vi "Train Approach.vi"(3 "Cycle State In":T1) -> (0 "Cycle State Out":T1)   [LabVIEW 2020]
uses:
  Reset.ctl
  Cycle Status.ctl
  Cycle Enum.ctl
  Grade Gate.ctl
  Global Indicators.vi
panel:
  out "Cycle Status":T2
  in  "Reset":T3
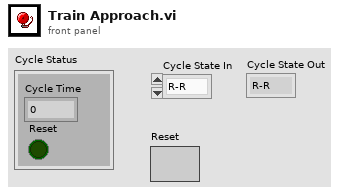
[diagram p1: front panel]
types:
  T1 = typedef "Cycle Enum.ctl" = enum16{"R-R", "NS Left G", "NS Left Y", "NS Straight G", "NS Straight Y", "r-r", "WE Left G", "WE Left Y", "WE Straight G", "WE Straight Y", "N All G", "S All G", "W All G", "E All G", "Gate Up", "Gate Mid", "Blink 1", "End Train", "Blink 2"}
  T2 = typedef "Cycle Status.ctl" = cluster{"Cycle Time":dbl, "Reset":bool}
  T3 = typedef "Reset.ctl" = bool
  T4 = typedef "Grade Gate.ctl" = cluster{"UP 2":bool, "Pivot":bool, "UP 3":bool, "UP 4":bool, "UP 5":bool, "UP 6":bool, "DOWN 2":bool, "DOWN 3":bool, "DOWN 4":bool, "DOWN 5":bool, "DOWN 6":bool, "DOWN 7":bool, "DOWN 8":bool, "SIDE 2":bool, "SIDE 3":bool, "SIDE 4":bool, "SIDE 5":bool, "Blinky 2":bool, "Blinky 1":bool}
  T5 = typedef "Traffic Signal.ctl" = cluster{"Red Light":bool, "Yellow Light":bool, "Green Light":bool, "Yellow Turn":bool, "Green Turn":bool}
  T6 = typedef "PedX Signal.ctl" = cluster{"PedX Walk":bool, "PedX Stop":bool}
  T7 = enum16{"R-R", "NS Left G", "NS Left Y", "NS Straight G", "NS Straight Y", "r-r", "WE Left G", "WE Left Y", "WE Straight G", "WE Straight Y"}
  T8 = enum16{"R-R", "NS Left G", "NS Left Y", "NS Straight G", "NS Straight Y"}
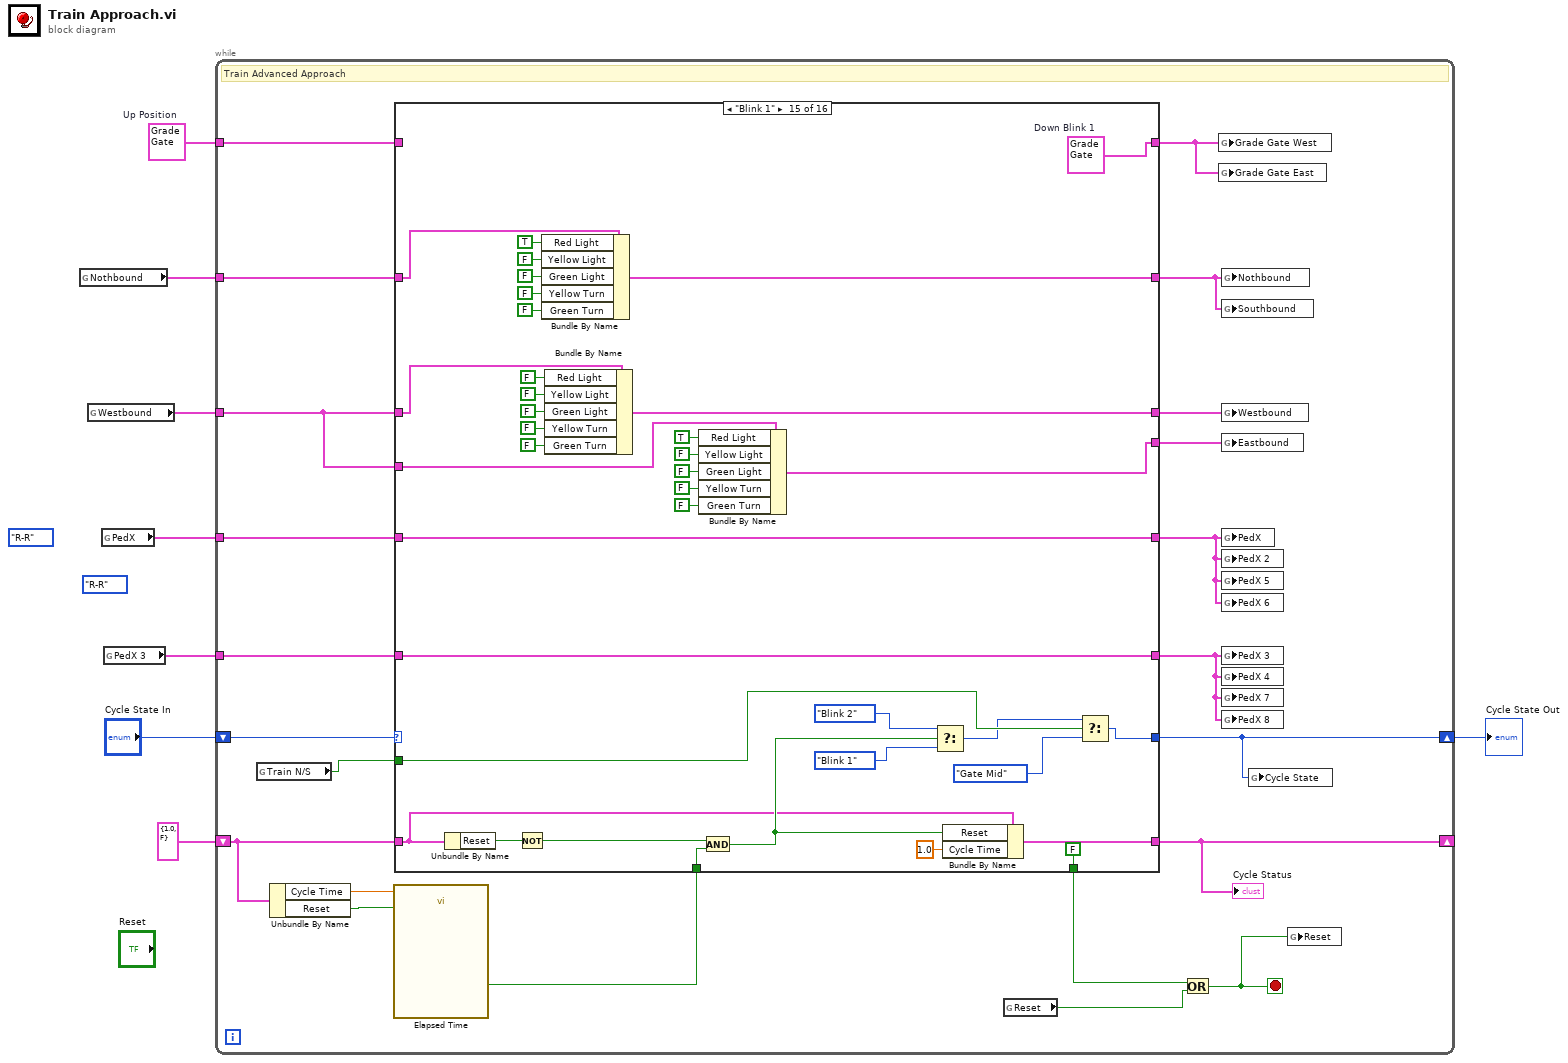
[diagram p0: block diagram]
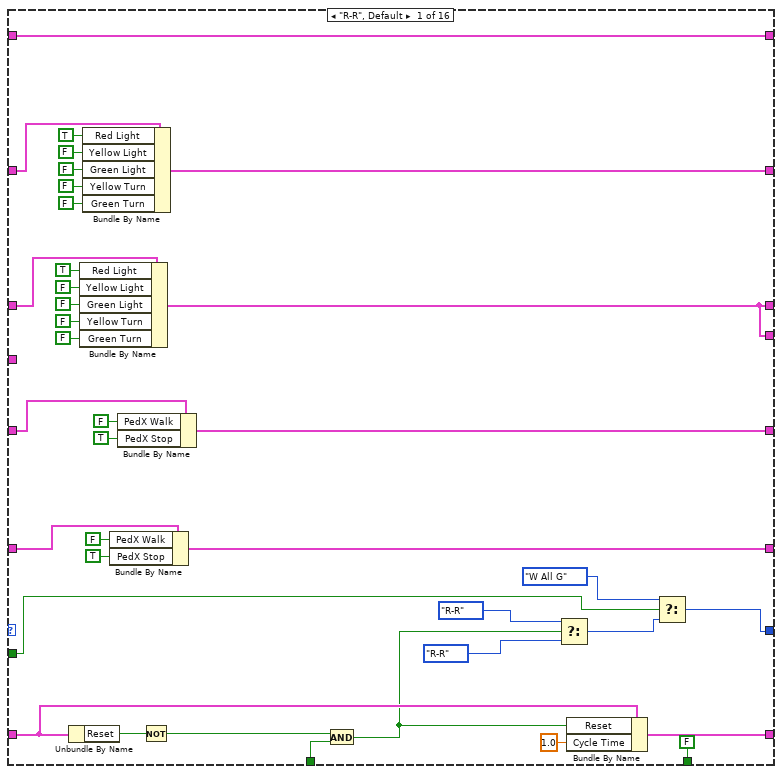
[diagram p2: hidden frame]
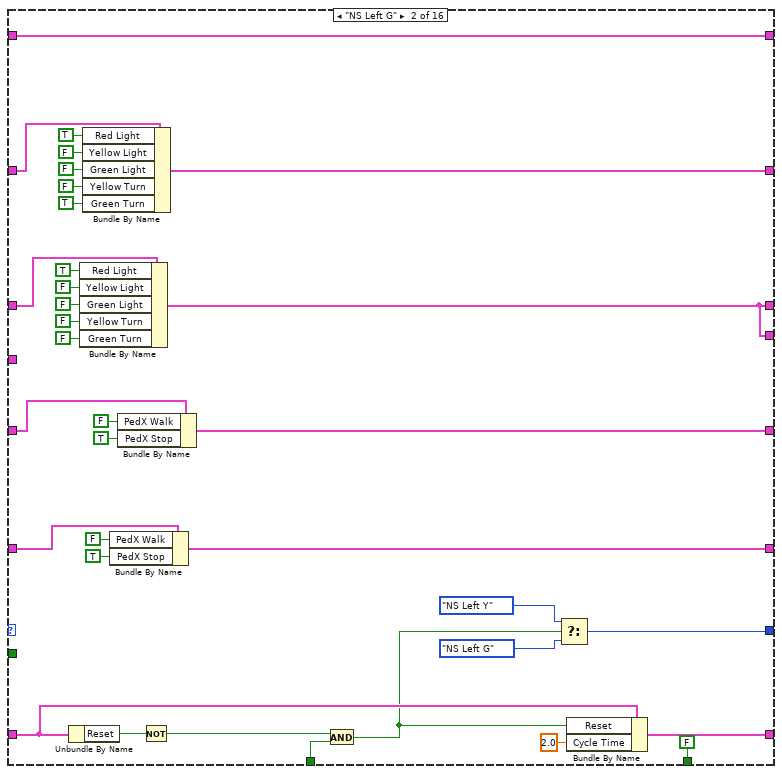
[diagram p3: hidden frame]
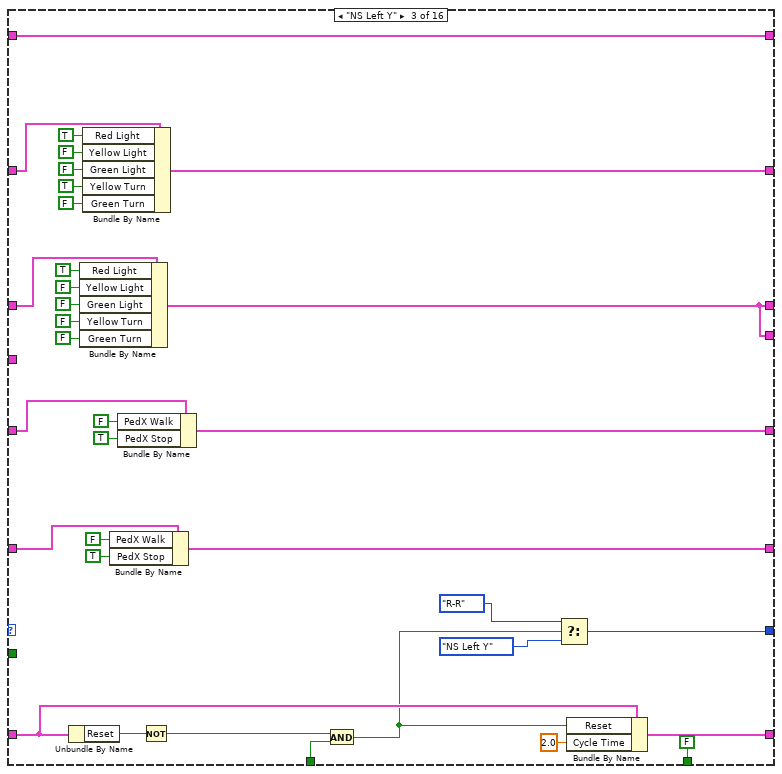
[diagram p4: hidden frame]
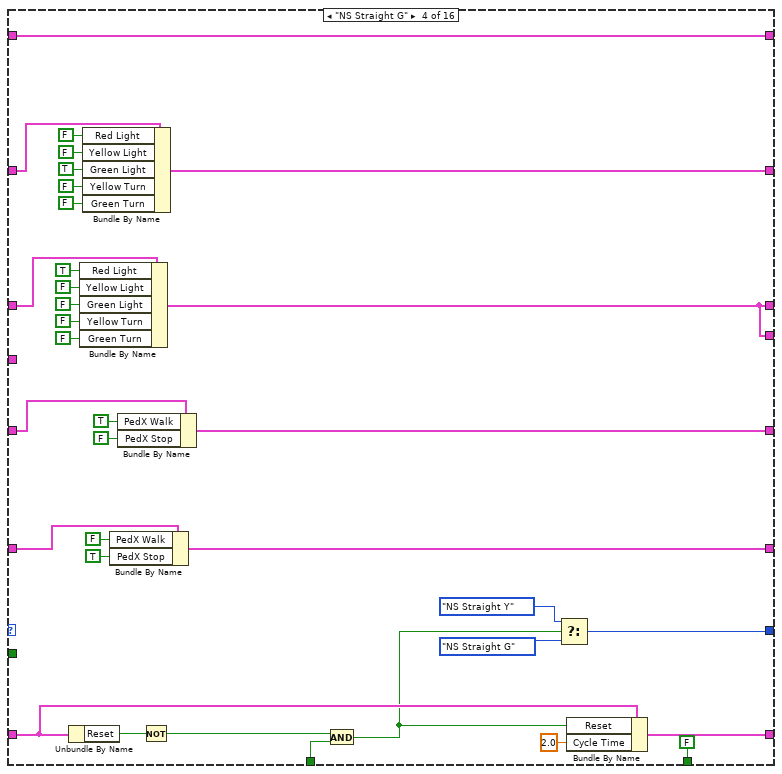
[diagram p5: hidden frame]
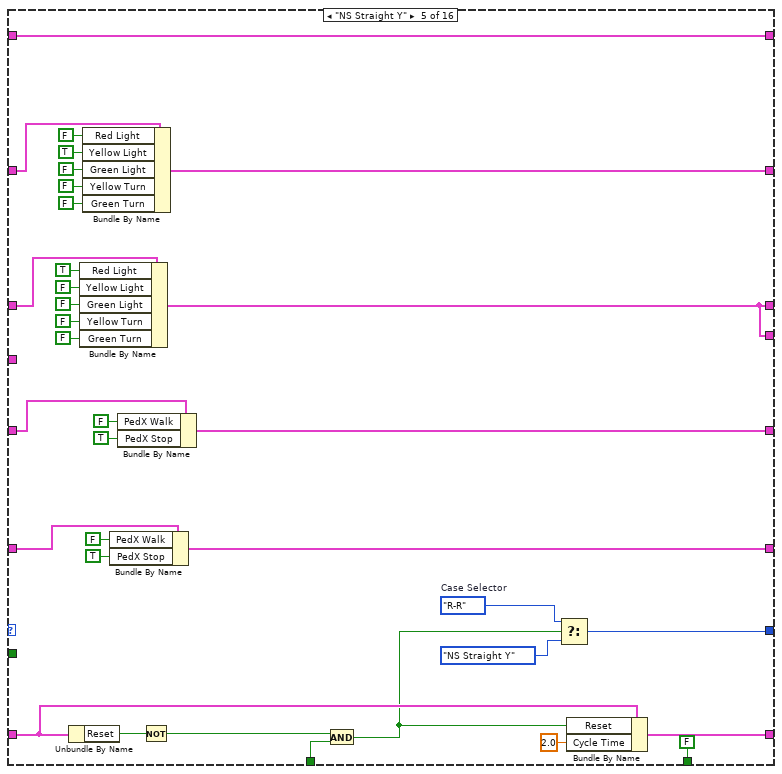
[diagram p6: hidden frame]
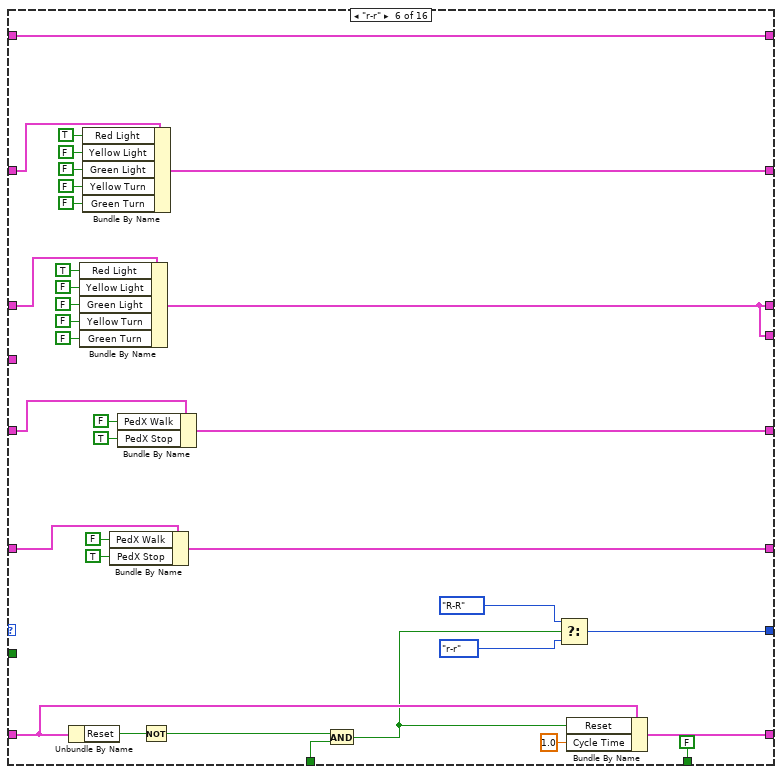
[diagram p7: hidden frame]
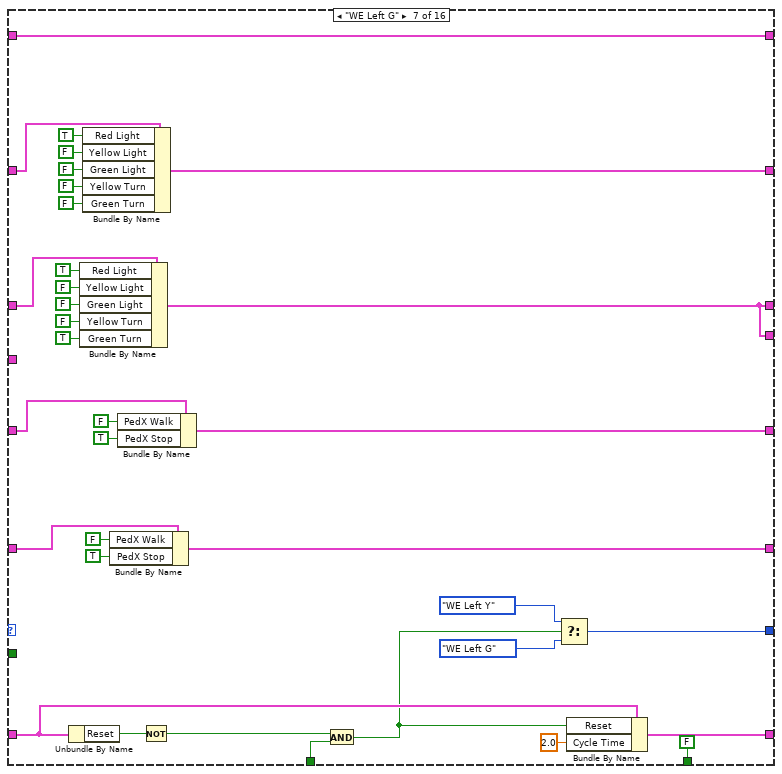
[diagram p8: hidden frame]
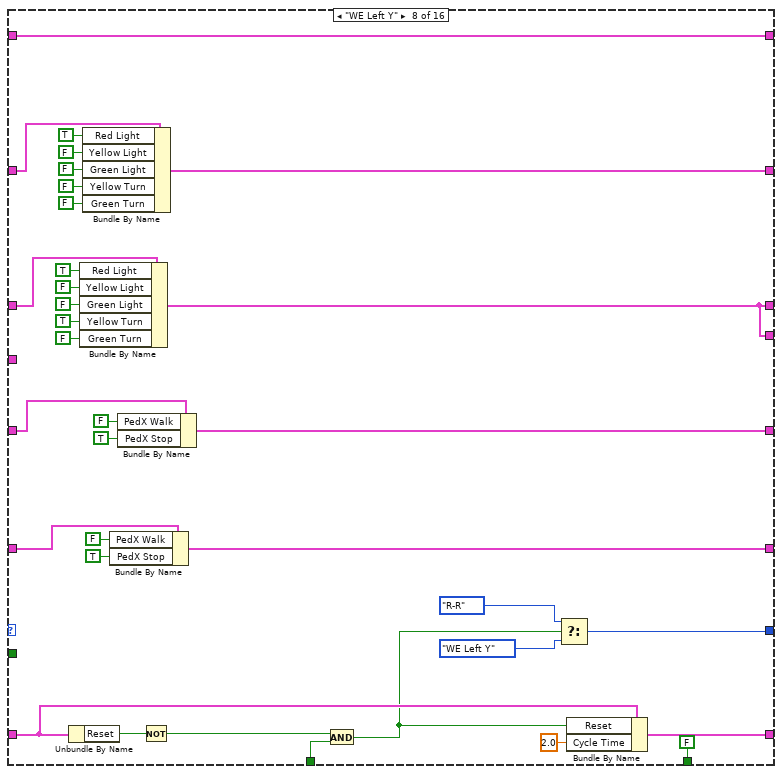
[diagram p9: hidden frame]
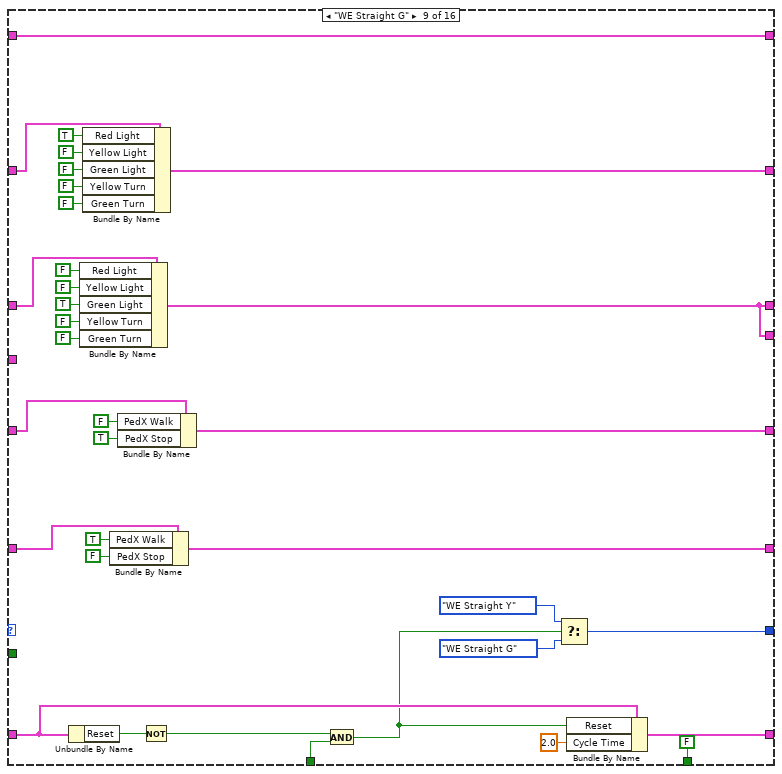
[diagram p10: hidden frame]
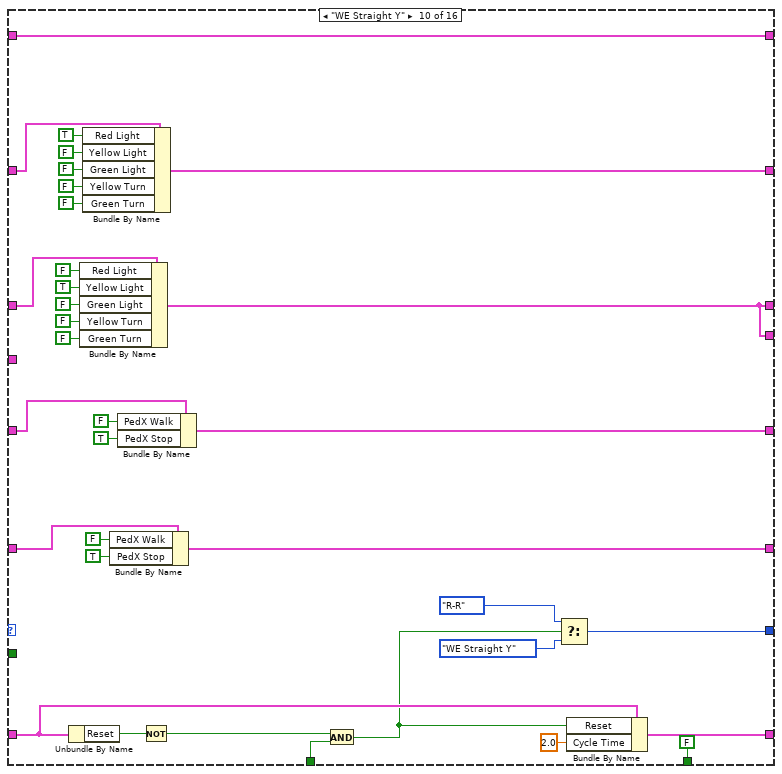
[diagram p11: hidden frame]
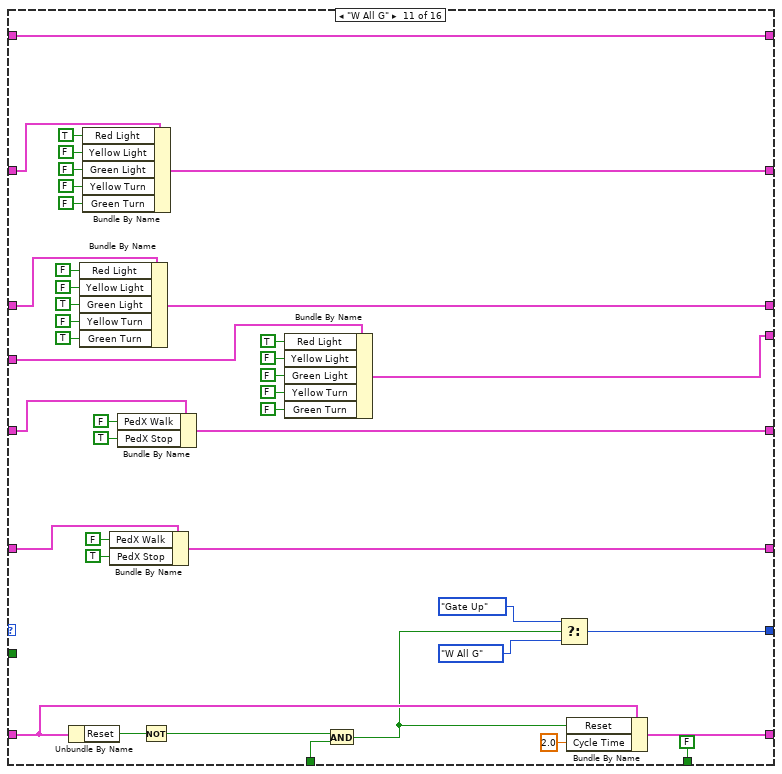
[diagram p12: hidden frame]
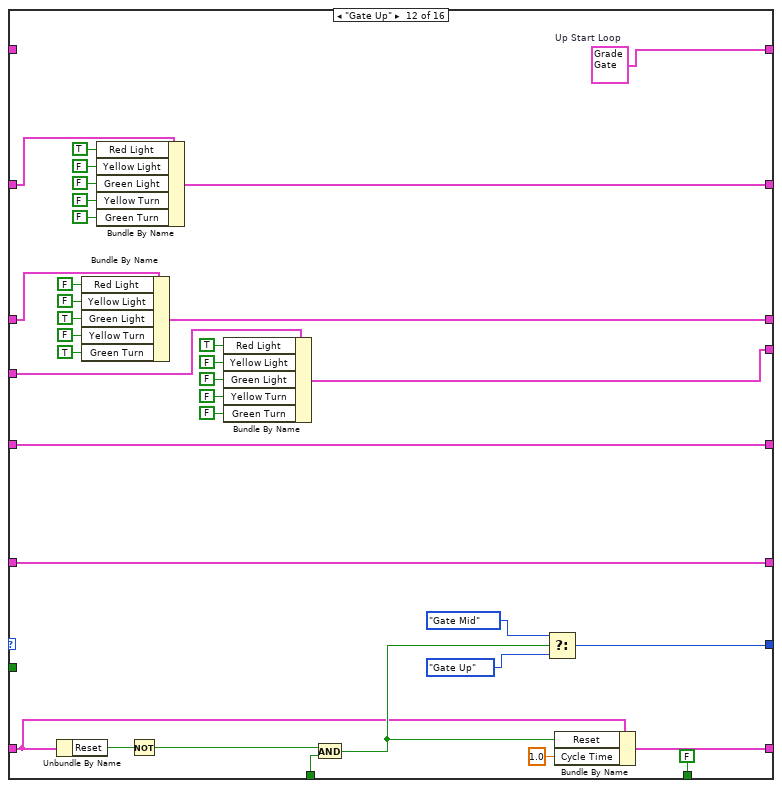
[diagram p13: hidden frame]
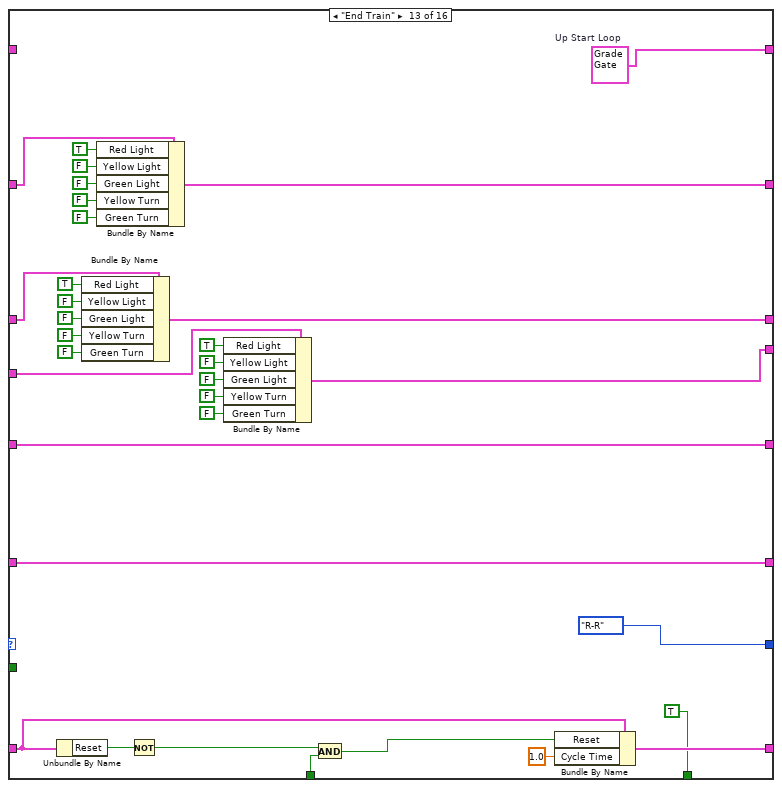
[diagram p14: hidden frame]
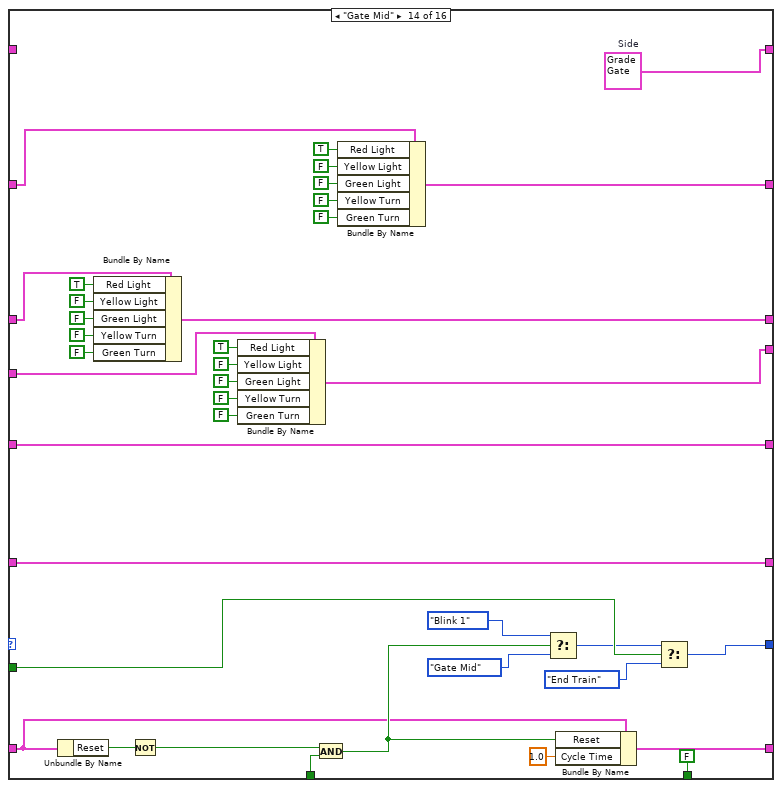
[diagram p15: hidden frame]
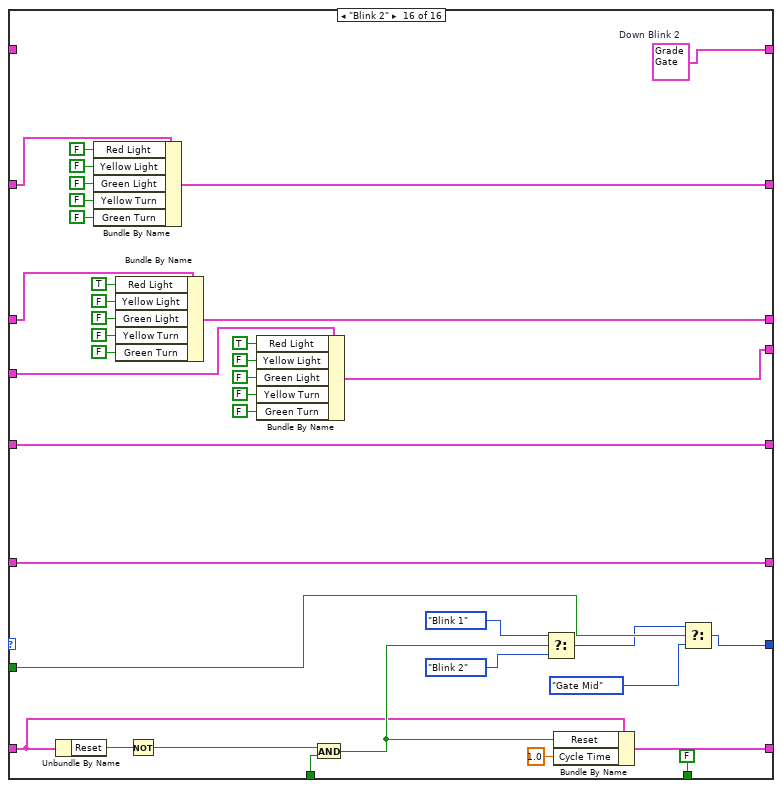
[diagram p16: hidden frame]
diagram:
  (unwired) Cycle_Enum."R-R" ("Cycle State In")
  (unwired) Cycle_Enum."R-R" ("Cycle State In")
  w8 = T4 {"UP 2"=FALSE, "Pivot"=FALSE, "UP 3"=TRUE, "UP 4"=FALSE, "UP 5"=FALSE, "UP 6"=FALSE, "DOWN 2"=FALSE, "DOWN 3"=FALSE, "DOWN 4"=FALSE, "DOWN 5"=FALSE, "DOWN 6"=FALSE, "DOWN 7"=FALSE, "DOWN 8"=FALSE, "SIDE 2"=FALSE, "SIDE 3"=FALSE, "SIDE 4"=FALSE, "SIDE 5"=FALSE, "Blinky 2"=FALSE, "Blinky 1"=FALSE}  # Up Position
  n1 = global read "Global Indicators.vi" "Nothbound"() -> (w6:T5)
  n2 = global read "Global Indicators.vi" "Westbound"() -> (w5:T5)
  n3 = global read "Global Indicators.vi" "PedX"() -> (w4:T6)
  n4 = global read "Global Indicators.vi" "PedX 3"() -> (w3:T6)
  n5 = while {
    shift-right: [w15] -> w1
    shift-left: "Cycle State In" -> [w17]
    tunnel: w8 -> [w26]
    tunnel: w5 -> [w14]
    tunnel: w6 -> [w25]
    tunnel: w4 -> [w24]
    tunnel: w3 -> [w23]
    shift-right: [w16] -> _
    shift-left: T2 {"Cycle Time"=1.0, "Reset"=FALSE} ("Cycle Status") -> [w22]
    stop <- w9 stop-if-true
    # "Train Advanced Approach"
    n6 = global read "Global Indicators.vi" "Train N/S"() -> (w10:bool)
    n7 = Unbundle By Name(w22) -> ("Cycle Time"=w30:dbl, "Reset"=w29:bool)
    n8 = call "Elapsed Time"("Time Target (s)"=w30, "Reset"=w29) -> ("Time has Elapsed"=w28:bool)  [unwired: 10 in, 7 out]
    n9 = case shown="\"Blink 1\"" w17 {
      tunnel: [w67 w101 w135 w169 w203 w237 w271 w305 w339 w373 w414 w449 w482 w520 w558 w596] -> w27
      tunnel: w26 -> [w67 w101 w135 w169 w203 w237 w271 w305 w339 w373 w414 _ _ _ _ _]
      tunnel: [w60 w94 w128 w162 w196 w230 w264 w298 w332 w366 w407 w445 w478 w518 w556 w592] -> w21
      tunnel: w25 -> [w66 w100 w134 w168 w202 w236 w270 w304 w338 w372 w413 w446 w479 w519 w557 w593]
      tunnel: [w37 w69 w103 w137 w171 w205 w239 w273 w307 w341 w393 w438 w471 w511 w549 w585] -> w20
      tunnel: w14 -> [w48 w81 w114 w147 w183 w217 w251 w285 w319 w353 w394 w439 w472 w512 w550 w586]
      tunnel: [w56 w90 w124 w158 w192 w226 w260 w294 w328 w362 w403 w448 w481 w505 w543 w595] -> w19
      tunnel: w24 -> [w59 w93 w127 w161 w195 w229 w263 w297 w331 w365 w406 w448 w481 w505 w543 w595]
      tunnel: w23 -> [w39 w72 w105 w138 w174 w208 w242 w276 w310 w344 w384 w447 w480 w504 w542 w594]
      tunnel: [w40 w73 w106 w139 w175 w209 w243 w277 w311 w345 w385 w447 w480 w504 w542 w594] -> w18
      tunnel: [w52 w85 w118 w151 w187 w221 w255 w289 w323 w357 w398 w418 w454 w490 w528 w566] -> w16
      tunnel: w22 -> [w51 w84 w117 w150 w186 w220 w254 w288 w322 w356 w397 w417 w453 w489 w527 w565]
      tunnel: [w33 w86 w120 w154 w188 w222 w256 w290 w324 w358 w399 w419 Cycle_Enum."R-R" ("Cycle State In") w487 w525 w562] -> w15
      tunnel: w28 -> [w53 w87 w121 w155 w189 w223 w257 w291 w325 w359 w400 w416 w452 w488 w526 w564]
      tunnel: w14 -> [_ _ _ _ _ _ _ _ _ _ w383 w432 w465 w503 w541 w579]
      tunnel: [w37 w69 w103 w137 w171 w205 w239 w273 w307 w341 w377 w431 w464 w502 w540 w578] -> w13
      tunnel: w10 -> [w32 _ _ _ _ _ _ _ _ _ _ _ _ w486 w524 w563]
      tunnel: [FALSE FALSE FALSE FALSE FALSE FALSE FALSE FALSE FALSE FALSE FALSE FALSE TRUE FALSE FALSE FALSE] -> w11
      frame "R-R", Default {
        n10 = Unbundle By Name(w51) -> ("Reset"=w55:bool)
        n11 = Bundle By Name(cluster=w48, "Red Light"=TRUE, "Yellow Light"=FALSE, "Green Light"=FALSE, "Yellow Turn"=FALSE, "Green Turn"=FALSE) -> (w37:T5)
        n12 = Bundle By Name(cluster=w66, "Red Light"=TRUE, "Yellow Light"=FALSE, "Green Light"=FALSE, "Yellow Turn"=FALSE, "Green Turn"=FALSE) -> (w60:T5)
        n13 = Bundle By Name(cluster=w39, "PedX Walk"=FALSE, "PedX Stop"=TRUE) -> (w40:T6)
        n14 = Bundle By Name(cluster=w59, "PedX Walk"=FALSE, "PedX Stop"=TRUE) -> (w56:T6)
        n15 = Not(x=w55) -> (.not. x?=w54:bool)
        n16 = And(x=w54, y=w53) -> (x .and. y?=w50:bool)
        n17 = Select(t=Cycle_Enum."R-R" ("Cycle State In"), s=w50, f=Cycle_Enum."R-R" ("Cycle State In")) -> (s? t:f=w34:T1)
        n18 = Bundle By Name(cluster=w51, "Reset"=w50, "Cycle Time"=1.0) -> (w52:T2)
        n19 = Select(t=Cycle_Enum."W All G" ("Cycle State In"), s=w32, f=w34) -> (s? t:f=w33:T1)
      }
      frame "NS Left G" {
        n20 = Unbundle By Name(w84) -> ("Reset"=w89:bool)
        n21 = Bundle By Name(cluster=w81, "Red Light"=TRUE, "Yellow Light"=FALSE, "Green Light"=FALSE, "Yellow Turn"=FALSE, "Green Turn"=FALSE) -> (w69:T5)
        n22 = Bundle By Name(cluster=w100, "Red Light"=TRUE, "Yellow Light"=FALSE, "Green Light"=FALSE, "Yellow Turn"=FALSE, "Green Turn"=TRUE) -> (w94:T5)
        n23 = Bundle By Name(cluster=w72, "PedX Walk"=FALSE, "PedX Stop"=TRUE) -> (w73:T6)
        n24 = Bundle By Name(cluster=w93, "PedX Walk"=FALSE, "PedX Stop"=TRUE) -> (w90:T6)
        n25 = Not(x=w89) -> (.not. x?=w88:bool)
        n26 = And(x=w88, y=w87) -> (x .and. y?=w83:bool)
        n27 = Select(t=T7."NS Left Y" ("Case Selector"), s=w83, f=T7."NS Left G" ("Case Selector")) -> (s? t:f=w86:T7)
        n28 = Bundle By Name(cluster=w84, "Reset"=w83, "Cycle Time"=2.0) -> (w85:T2)
      }
      frame "NS Left Y" {
        n29 = Unbundle By Name(w117) -> ("Reset"=w123:bool)
        n30 = Bundle By Name(cluster=w114, "Red Light"=TRUE, "Yellow Light"=FALSE, "Green Light"=FALSE, "Yellow Turn"=FALSE, "Green Turn"=FALSE) -> (w103:T5)
        n31 = Bundle By Name(cluster=w134, "Red Light"=TRUE, "Yellow Light"=FALSE, "Green Light"=FALSE, "Yellow Turn"=TRUE, "Green Turn"=FALSE) -> (w128:T5)
        n32 = Bundle By Name(cluster=w105, "PedX Walk"=FALSE, "PedX Stop"=TRUE) -> (w106:T6)
        n33 = Bundle By Name(cluster=w127, "PedX Walk"=FALSE, "PedX Stop"=TRUE) -> (w124:T6)
        n34 = Not(x=w123) -> (.not. x?=w122:bool)
        n35 = And(x=w122, y=w121) -> (x .and. y?=w116:bool)
        n36 = Select(t=Cycle_Enum."R-R" ("Cycle State In"), s=w116, f=T8."NS Left Y" ("Case Selector")) -> (s? t:f=w120:T1)
        n37 = Bundle By Name(cluster=w117, "Reset"=w116, "Cycle Time"=2.0) -> (w118:T2)
      }
      frame "NS Straight G" {
        n38 = Unbundle By Name(w150) -> ("Reset"=w157:bool)
        n39 = Bundle By Name(cluster=w147, "Red Light"=TRUE, "Yellow Light"=FALSE, "Green Light"=FALSE, "Yellow Turn"=FALSE, "Green Turn"=FALSE) -> (w137:T5)
        n40 = Bundle By Name(cluster=w168, "Red Light"=FALSE, "Yellow Light"=FALSE, "Green Light"=TRUE, "Yellow Turn"=FALSE, "Green Turn"=FALSE) -> (w162:T5)
        n41 = Bundle By Name(cluster=w138, "PedX Walk"=FALSE, "PedX Stop"=TRUE) -> (w139:T6)
        n42 = Bundle By Name(cluster=w161, "PedX Walk"=TRUE, "PedX Stop"=FALSE) -> (w158:T6)
        n43 = Not(x=w157) -> (.not. x?=w156:bool)
        n44 = And(x=w156, y=w155) -> (x .and. y?=w149:bool)
        n45 = Select(t=T8."NS Straight Y" ("Case Selector"), s=w149, f=T8."NS Straight G" ("Case Selector")) -> (s? t:f=w154:T8)
        n46 = Bundle By Name(cluster=w150, "Reset"=w149, "Cycle Time"=2.0) -> (w151:T2)
      }
      frame "NS Straight Y" {
        w173 = T7."R-R"  # Case Selector
        n47 = Unbundle By Name(w186) -> ("Reset"=w191:bool)
        n48 = Bundle By Name(cluster=w183, "Red Light"=TRUE, "Yellow Light"=FALSE, "Green Light"=FALSE, "Yellow Turn"=FALSE, "Green Turn"=FALSE) -> (w171:T5)
        n49 = Bundle By Name(cluster=w202, "Red Light"=FALSE, "Yellow Light"=TRUE, "Green Light"=FALSE, "Yellow Turn"=FALSE, "Green Turn"=FALSE) -> (w196:T5)
        n50 = Bundle By Name(cluster=w174, "PedX Walk"=FALSE, "PedX Stop"=TRUE) -> (w175:T6)
        n51 = Bundle By Name(cluster=w195, "PedX Walk"=FALSE, "PedX Stop"=TRUE) -> (w192:T6)
        n52 = Not(x=w191) -> (.not. x?=w190:bool)
        n53 = And(x=w190, y=w189) -> (x .and. y?=w185:bool)
        n54 = Select(t=w173, s=w185, f=T7."NS Straight Y" ("Case Selector")) -> (s? t:f=w188:T7)
        n55 = Bundle By Name(cluster=w186, "Reset"=w185, "Cycle Time"=2.0) -> (w187:T2)
      }
      frame "r-r" {
        n56 = Unbundle By Name(w220) -> ("Reset"=w225:bool)
        n57 = Bundle By Name(cluster=w217, "Red Light"=TRUE, "Yellow Light"=FALSE, "Green Light"=FALSE, "Yellow Turn"=FALSE, "Green Turn"=FALSE) -> (w205:T5)
        n58 = Bundle By Name(cluster=w236, "Red Light"=TRUE, "Yellow Light"=FALSE, "Green Light"=FALSE, "Yellow Turn"=FALSE, "Green Turn"=FALSE) -> (w230:T5)
        n59 = Bundle By Name(cluster=w208, "PedX Walk"=FALSE, "PedX Stop"=TRUE) -> (w209:T6)
        n60 = Bundle By Name(cluster=w229, "PedX Walk"=FALSE, "PedX Stop"=TRUE) -> (w226:T6)
        n61 = Not(x=w225) -> (.not. x?=w224:bool)
        n62 = And(x=w224, y=w223) -> (x .and. y?=w219:bool)
        n63 = Select(t=T7."R-R" ("Case Selector"), s=w219, f=T7."r-r" ("Case Selector")) -> (s? t:f=w222:T7)
        n64 = Bundle By Name(cluster=w220, "Reset"=w219, "Cycle Time"=1.0) -> (w221:T2)
      }
      frame "WE Left G" {
        n65 = Unbundle By Name(w254) -> ("Reset"=w259:bool)
        n66 = Bundle By Name(cluster=w251, "Red Light"=TRUE, "Yellow Light"=FALSE, "Green Light"=FALSE, "Yellow Turn"=FALSE, "Green Turn"=TRUE) -> (w239:T5)
        n67 = Bundle By Name(cluster=w270, "Red Light"=TRUE, "Yellow Light"=FALSE, "Green Light"=FALSE, "Yellow Turn"=FALSE, "Green Turn"=FALSE) -> (w264:T5)
        n68 = Bundle By Name(cluster=w242, "PedX Walk"=FALSE, "PedX Stop"=TRUE) -> (w243:T6)
        n69 = Bundle By Name(cluster=w263, "PedX Walk"=FALSE, "PedX Stop"=TRUE) -> (w260:T6)
        n70 = Not(x=w259) -> (.not. x?=w258:bool)
        n71 = And(x=w258, y=w257) -> (x .and. y?=w253:bool)
        n72 = Select(t=T7."WE Left Y" ("Case Selector"), s=w253, f=T7."WE Left G" ("Case Selector")) -> (s? t:f=w256:T7)
        n73 = Bundle By Name(cluster=w254, "Reset"=w253, "Cycle Time"=2.0) -> (w255:T2)
      }
      frame "WE Left Y" {
        n74 = Unbundle By Name(w288) -> ("Reset"=w293:bool)
        n75 = Bundle By Name(cluster=w285, "Red Light"=TRUE, "Yellow Light"=FALSE, "Green Light"=FALSE, "Yellow Turn"=TRUE, "Green Turn"=FALSE) -> (w273:T5)
        n76 = Bundle By Name(cluster=w304, "Red Light"=TRUE, "Yellow Light"=FALSE, "Green Light"=FALSE, "Yellow Turn"=FALSE, "Green Turn"=FALSE) -> (w298:T5)
        n77 = Bundle By Name(cluster=w276, "PedX Walk"=FALSE, "PedX Stop"=TRUE) -> (w277:T6)
        n78 = Bundle By Name(cluster=w297, "PedX Walk"=FALSE, "PedX Stop"=TRUE) -> (w294:T6)
        n79 = Not(x=w293) -> (.not. x?=w292:bool)
        n80 = And(x=w292, y=w291) -> (x .and. y?=w287:bool)
        n81 = Select(t=T7."R-R" ("Case Selector"), s=w287, f=T7."WE Left Y" ("Case Selector")) -> (s? t:f=w290:T7)
        n82 = Bundle By Name(cluster=w288, "Reset"=w287, "Cycle Time"=2.0) -> (w289:T2)
      }
      frame "WE Straight G" {
        n83 = Unbundle By Name(w322) -> ("Reset"=w327:bool)
        n84 = Bundle By Name(cluster=w319, "Red Light"=FALSE, "Yellow Light"=FALSE, "Green Light"=TRUE, "Yellow Turn"=FALSE, "Green Turn"=FALSE) -> (w307:T5)
        n85 = Bundle By Name(cluster=w338, "Red Light"=TRUE, "Yellow Light"=FALSE, "Green Light"=FALSE, "Yellow Turn"=FALSE, "Green Turn"=FALSE) -> (w332:T5)
        n86 = Bundle By Name(cluster=w310, "PedX Walk"=TRUE, "PedX Stop"=FALSE) -> (w311:T6)
        n87 = Bundle By Name(cluster=w331, "PedX Walk"=FALSE, "PedX Stop"=TRUE) -> (w328:T6)
        n88 = Not(x=w327) -> (.not. x?=w326:bool)
        n89 = And(x=w326, y=w325) -> (x .and. y?=w321:bool)
        n90 = Select(t=T7."WE Straight Y" ("Case Selector"), s=w321, f=T7."WE Straight G" ("Case Selector")) -> (s? t:f=w324:T7)
        n91 = Bundle By Name(cluster=w322, "Reset"=w321, "Cycle Time"=2.0) -> (w323:T2)
      }
      frame "WE Straight Y" {
        n92 = Unbundle By Name(w356) -> ("Reset"=w361:bool)
        n93 = Bundle By Name(cluster=w353, "Red Light"=FALSE, "Yellow Light"=TRUE, "Green Light"=FALSE, "Yellow Turn"=FALSE, "Green Turn"=FALSE) -> (w341:T5)
        n94 = Bundle By Name(cluster=w372, "Red Light"=TRUE, "Yellow Light"=FALSE, "Green Light"=FALSE, "Yellow Turn"=FALSE, "Green Turn"=FALSE) -> (w366:T5)
        n95 = Bundle By Name(cluster=w344, "PedX Walk"=FALSE, "PedX Stop"=TRUE) -> (w345:T6)
        n96 = Bundle By Name(cluster=w365, "PedX Walk"=FALSE, "PedX Stop"=TRUE) -> (w362:T6)
        n97 = Not(x=w361) -> (.not. x?=w360:bool)
        n98 = And(x=w360, y=w359) -> (x .and. y?=w355:bool)
        n99 = Select(t=T7."R-R" ("Case Selector"), s=w355, f=T7."WE Straight Y" ("Case Selector")) -> (s? t:f=w358:T7)
        n100 = Bundle By Name(cluster=w356, "Reset"=w355, "Cycle Time"=2.0) -> (w357:T2)
      }
      frame "W All G" {
        n101 = Unbundle By Name(w397) -> ("Reset"=w402:bool)
        n102 = Bundle By Name(cluster=w394, "Red Light"=FALSE, "Yellow Light"=FALSE, "Green Light"=TRUE, "Yellow Turn"=FALSE, "Green Turn"=TRUE) -> (w393:T5)
        n103 = Bundle By Name(cluster=w413, "Red Light"=TRUE, "Yellow Light"=FALSE, "Green Light"=FALSE, "Yellow Turn"=FALSE, "Green Turn"=FALSE) -> (w407:T5)
        n104 = Bundle By Name(cluster=w384, "PedX Walk"=FALSE, "PedX Stop"=TRUE) -> (w385:T6)
        n105 = Bundle By Name(cluster=w406, "PedX Walk"=FALSE, "PedX Stop"=TRUE) -> (w403:T6)
        n106 = Not(x=w402) -> (.not. x?=w401:bool)
        n107 = Bundle By Name(cluster=w383, "Red Light"=TRUE, "Yellow Light"=FALSE, "Green Light"=FALSE, "Yellow Turn"=FALSE, "Green Turn"=FALSE) -> (w377:T5)
        n108 = And(x=w401, y=w400) -> (x .and. y?=w396:bool)
        n109 = Select(t=Cycle_Enum."Gate Up" ("Cycle State In"), s=w396, f=Cycle_Enum."W All G" ("Cycle State In")) -> (s? t:f=w399:T1)
        n110 = Bundle By Name(cluster=w397, "Reset"=w396, "Cycle Time"=2.0) -> (w398:T2)
      }
      frame "Gate Up" {
        w449 = T4 {"UP 2"=FALSE, "Pivot"=FALSE, "UP 3"=TRUE, "UP 4"=FALSE, "UP 5"=FALSE, "UP 6"=FALSE, "DOWN 2"=FALSE, "DOWN 3"=FALSE, "DOWN 4"=FALSE, "DOWN 5"=FALSE, "DOWN 6"=FALSE, "DOWN 7"=FALSE, "DOWN 8"=FALSE, "SIDE 2"=FALSE, "SIDE 3"=FALSE, "SIDE 4"=FALSE, "SIDE 5"=FALSE, "Blinky 2"=FALSE, "Blinky 1"=FALSE}  # Up Start Loop
        n111 = Unbundle By Name(w417) -> ("Reset"=w425:bool)
        n112 = Bundle By Name(cluster=w439, "Red Light"=FALSE, "Yellow Light"=FALSE, "Green Light"=TRUE, "Yellow Turn"=FALSE, "Green Turn"=TRUE) -> (w438:T5)
        n113 = Bundle By Name(cluster=w446, "Red Light"=TRUE, "Yellow Light"=FALSE, "Green Light"=FALSE, "Yellow Turn"=FALSE, "Green Turn"=FALSE) -> (w445:T5)
        n114 = Not(x=w425) -> (.not. x?=w424:bool)
        n115 = Bundle By Name(cluster=w432, "Red Light"=TRUE, "Yellow Light"=FALSE, "Green Light"=FALSE, "Yellow Turn"=FALSE, "Green Turn"=FALSE) -> (w431:T5)
        n116 = And(x=w424, y=w416) -> (x .and. y?=w423:bool)
        n117 = Select(t=Cycle_Enum."Gate Mid" ("Cycle State In"), s=w423, f=Cycle_Enum."Gate Up" ("Cycle State In")) -> (s? t:f=w419:T1)
        n118 = Bundle By Name(cluster=w417, "Reset"=w423, "Cycle Time"=1.0) -> (w418:T2)
      }
      frame "End Train" {
        w482 = T4 {"UP 2"=FALSE, "Pivot"=FALSE, "UP 3"=TRUE, "UP 4"=FALSE, "UP 5"=FALSE, "UP 6"=FALSE, "DOWN 2"=FALSE, "DOWN 3"=FALSE, "DOWN 4"=FALSE, "DOWN 5"=FALSE, "DOWN 6"=FALSE, "DOWN 7"=FALSE, "DOWN 8"=FALSE, "SIDE 2"=FALSE, "SIDE 3"=FALSE, "SIDE 4"=FALSE, "SIDE 5"=FALSE, "Blinky 2"=FALSE, "Blinky 1"=FALSE}  # Up Start Loop
        n119 = Unbundle By Name(w453) -> ("Reset"=w458:bool)
        n120 = Bundle By Name(cluster=w472, "Red Light"=TRUE, "Yellow Light"=FALSE, "Green Light"=FALSE, "Yellow Turn"=FALSE, "Green Turn"=FALSE) -> (w471:T5)
        n121 = Bundle By Name(cluster=w479, "Red Light"=TRUE, "Yellow Light"=FALSE, "Green Light"=FALSE, "Yellow Turn"=FALSE, "Green Turn"=FALSE) -> (w478:T5)
        n122 = Not(x=w458) -> (.not. x?=w457:bool)
        n123 = Bundle By Name(cluster=w465, "Red Light"=TRUE, "Yellow Light"=FALSE, "Green Light"=FALSE, "Yellow Turn"=FALSE, "Green Turn"=FALSE) -> (w464:T5)
        n124 = And(x=w457, y=w452) -> (x .and. y?=w456:bool)
        n125 = Bundle By Name(cluster=w453, "Reset"=w456, "Cycle Time"=1.0) -> (w454:T2)
      }
      frame "Gate Mid" {
        w520 = T4 {"UP 2"=TRUE, "Pivot"=FALSE, "UP 3"=FALSE, "UP 4"=TRUE, "UP 5"=TRUE, "UP 6"=TRUE, "DOWN 2"=FALSE, "DOWN 3"=FALSE, "DOWN 4"=FALSE, "DOWN 5"=FALSE, "DOWN 6"=FALSE, "DOWN 7"=FALSE, "DOWN 8"=FALSE, "SIDE 2"=TRUE, "SIDE 3"=TRUE, "SIDE 4"=TRUE, "SIDE 5"=TRUE, "Blinky 2"=FALSE, "Blinky 1"=FALSE}  # Side
        n126 = Unbundle By Name(w489) -> ("Reset"=w496:bool)
        n127 = Bundle By Name(cluster=w512, "Red Light"=TRUE, "Yellow Light"=FALSE, "Green Light"=FALSE, "Yellow Turn"=FALSE, "Green Turn"=FALSE) -> (w511:T5)
        n128 = Not(x=w496) -> (.not. x?=w495:bool)
        n129 = Bundle By Name(cluster=w503, "Red Light"=TRUE, "Yellow Light"=FALSE, "Green Light"=FALSE, "Yellow Turn"=FALSE, "Green Turn"=FALSE) -> (w502:T5)
        n130 = And(x=w495, y=w488) -> (x .and. y?=w494:bool)
        n131 = Bundle By Name(cluster=w519, "Red Light"=TRUE, "Yellow Light"=FALSE, "Green Light"=FALSE, "Yellow Turn"=FALSE, "Green Turn"=FALSE) -> (w518:T5)
        n132 = Select(t=Cycle_Enum."Blink 1" ("Cycle State In"), s=w494, f=Cycle_Enum."Gate Mid" ("Cycle State In")) -> (s? t:f=w485:T1)
        n133 = Bundle By Name(cluster=w489, "Reset"=w494, "Cycle Time"=1.0) -> (w490:T2)
        n134 = Select(t=w485, s=w486, f=Cycle_Enum."End Train" ("Cycle State In")) -> (s? t:f=w487:T1)
      }
      frame "Blink 1" {
        w558 = T4 {"UP 2"=TRUE, "Pivot"=FALSE, "UP 3"=FALSE, "UP 4"=TRUE, "UP 5"=TRUE, "UP 6"=TRUE, "DOWN 2"=TRUE, "DOWN 3"=TRUE, "DOWN 4"=TRUE, "DOWN 5"=TRUE, "DOWN 6"=TRUE, "DOWN 7"=FALSE, "DOWN 8"=TRUE, "SIDE 2"=FALSE, "SIDE 3"=FALSE, "SIDE 4"=FALSE, "SIDE 5"=FALSE, "Blinky 2"=TRUE, "Blinky 1"=FALSE}  # Down Blink 1
        n135 = Unbundle By Name(w527) -> ("Reset"=w534:bool)
        n136 = Not(x=w534) -> (.not. x?=w533:bool)
        n137 = Bundle By Name(cluster=w557, "Red Light"=TRUE, "Yellow Light"=FALSE, "Green Light"=FALSE, "Yellow Turn"=FALSE, "Green Turn"=FALSE) -> (w556:T5)
        n138 = Bundle By Name(cluster=w550, "Red Light"=FALSE, "Yellow Light"=FALSE, "Green Light"=FALSE, "Yellow Turn"=FALSE, "Green Turn"=FALSE) -> (w549:T5)
        n139 = Bundle By Name(cluster=w541, "Red Light"=TRUE, "Yellow Light"=FALSE, "Green Light"=FALSE, "Yellow Turn"=FALSE, "Green Turn"=FALSE) -> (w540:T5)
        n140 = And(x=w533, y=w526) -> (x .and. y?=w532:bool)
        n141 = Select(t=Cycle_Enum."Blink 2" ("Cycle State In"), s=w532, f=Cycle_Enum."Blink 1" ("Cycle State In")) -> (s? t:f=w523:T1)
        n142 = Bundle By Name(cluster=w527, "Reset"=w532, "Cycle Time"=1.0) -> (w528:T2)
        n143 = Select(t=w523, s=w524, f=Cycle_Enum."Gate Mid" ("Cycle State In")) -> (s? t:f=w525:T1)
      }
      frame "Blink 2" {
        w596 = T4 {"UP 2"=TRUE, "Pivot"=FALSE, "UP 3"=FALSE, "UP 4"=TRUE, "UP 5"=TRUE, "UP 6"=TRUE, "DOWN 2"=TRUE, "DOWN 3"=TRUE, "DOWN 4"=TRUE, "DOWN 5"=TRUE, "DOWN 6"=TRUE, "DOWN 7"=TRUE, "DOWN 8"=FALSE, "SIDE 2"=FALSE, "SIDE 3"=FALSE, "SIDE 4"=FALSE, "SIDE 5"=FALSE, "Blinky 2"=FALSE, "Blinky 1"=TRUE}  # Down Blink 2
        n144 = Unbundle By Name(w565) -> ("Reset"=w572:bool)
        n145 = Bundle By Name(cluster=w593, "Red Light"=FALSE, "Yellow Light"=FALSE, "Green Light"=FALSE, "Yellow Turn"=FALSE, "Green Turn"=FALSE) -> (w592:T5)
        n146 = Bundle By Name(cluster=w586, "Red Light"=TRUE, "Yellow Light"=FALSE, "Green Light"=FALSE, "Yellow Turn"=FALSE, "Green Turn"=FALSE) -> (w585:T5)
        n147 = Not(x=w572) -> (.not. x?=w571:bool)
        n148 = Bundle By Name(cluster=w579, "Red Light"=TRUE, "Yellow Light"=FALSE, "Green Light"=FALSE, "Yellow Turn"=FALSE, "Green Turn"=FALSE) -> (w578:T5)
        n149 = And(x=w571, y=w564) -> (x .and. y?=w570:bool)
        n150 = Select(t=Cycle_Enum."Blink 1" ("Cycle State In"), s=w570, f=Cycle_Enum."Blink 2" ("Cycle State In")) -> (s? t:f=w561:T1)
        n151 = Bundle By Name(cluster=w565, "Reset"=w570, "Cycle Time"=1.0) -> (w566:T2)
        n152 = Select(t=w561, s=w563, f=Cycle_Enum."Gate Mid" ("Cycle State In")) -> (s? t:f=w562:T1)
      }
    }
    "Cycle Status" <- w16
    n153 = global read "Global Indicators.vi" "Reset"() -> (w12:T3)
    n154 = Or(x=w11, y=w12) -> (x .or. y?=w9:T3)
    n155 = global write "Global Indicators.vi" "Grade Gate West"(w27) -> ()
    n156 = global write "Global Indicators.vi" "Grade Gate East"(w27) -> ()
    n157 = global write "Global Indicators.vi" "Nothbound"(w21) -> ()
    n158 = global write "Global Indicators.vi" "Southbound"(w21) -> ()
    n159 = global write "Global Indicators.vi" "Westbound"(w20) -> ()
    n160 = global write "Global Indicators.vi" "Eastbound"(w13) -> ()
    n161 = global write "Global Indicators.vi" "PedX"(w19) -> ()
    n162 = global write "Global Indicators.vi" "PedX 2"(w19) -> ()
    n163 = global write "Global Indicators.vi" "PedX 5"(w19) -> ()
    n164 = global write "Global Indicators.vi" "PedX 6"(w19) -> ()
    n165 = global write "Global Indicators.vi" "PedX 3"(w18) -> ()
    n166 = global write "Global Indicators.vi" "PedX 4"(w18) -> ()
    n167 = global write "Global Indicators.vi" "PedX 7"(w18) -> ()
    n168 = global write "Global Indicators.vi" "PedX 8"(w18) -> ()
    n169 = global write "Global Indicators.vi" "Cycle State"(w15) -> ()
    n170 = global write "Global Indicators.vi" "Reset"(w9) -> ()
  }
  "Cycle State Out" <- w1
